vi "Initialize ReadWrite Data.vi"(7 "Name":string, 8 "error in (no error)":errorcluster, 10 "Hardware Output Refs":T1[](array[typedef]) format="%.0x", 11 "Device Ref":T1 format="%.0x") -> (0 "error out":errorcluster, 2 "ReadWrite Data":T2 {"Pairs"."Chan Refs" format="%.0x"}, 3 "Device Ref out":T1=18446744073709551615 format="%.0x")   [LabVIEW 2013, in "FPGA Addon Engine.lvlib" / "Inline Async API.lvlib"]
uses:
  Inline Async API.lvlib
  Controls/ReadWrite Data.ctl
  <vilib>/NI Veristand/Custom Device API/Data Reference.ctl
  <vilib>/NI Veristand/Custom Device API/Custom Device Item Ref.ctl
  <vilib>/NI Veristand/Custom Device API/Data Access Type.ctl
  <vilib>/NI VeriStand/Custom Device API/Custom Device API.lvlib
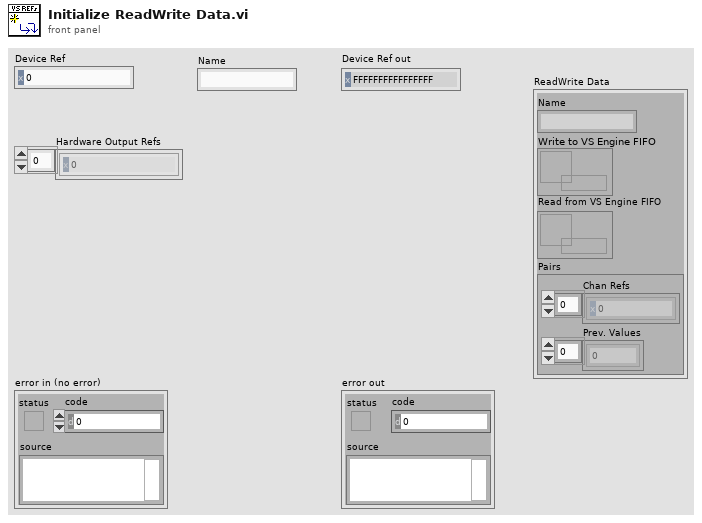
[diagram p1: front panel]
types:
  T1 = typedef "Custom Device API.lvlib/Custom Device Item Ref.ctl" = u64
  T2 = typedef "FPGA Addon Engine.lvlib/Inline Async API.lvlib/ReadWrite Data.ctl" = cluster{"Name":string, "Write to VS Engine FIFO":refnum<k33>, "Read from VS Engine FIFO":refnum<k33>, "Pairs":cluster{"Chan Refs":T3[], "Prev. Values":dbl[]}}
  T3 = typedef "Custom Device API.lvlib/Data Reference.ctl" = i32
  T4 = cluster{"read mode":enum16{"polling", "blocking"}, "write mode":enum16{"polling", "blocking"}}
  T5 = typedef "Custom Device API.lvlib/Data Access Type.ctl" = enum16{"Read", "Write"}
  T6 = typedef "Custom Device API.lvlib/Custom Device Item Info.ctl" = cluster{"Name":string, "Is Channel":bool, "GUID":string, "Is Waveform":bool}
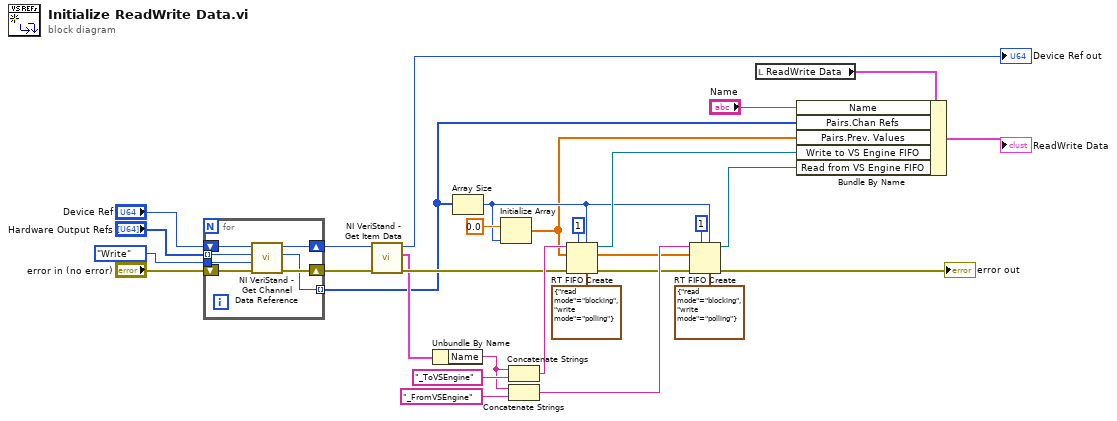
[diagram p0: block diagram]
diagram:
  n1 = for {
    tunnel: "Hardware Output Refs" -> [w32] mode=indexing
    tunnel: Data_Access_Type."Write" ("Access") -> [w31]
    shift-right: [w34] -> w9
    shift-left: "error in (no error)" -> [w35]
    shift-right: [w36] -> w7
    shift-left: "Device Ref" -> [w33]
    tunnel: [w30] -> w3 mode=indexing
    n2 = call <vilib>:"NI VeriStand - Get Channel Data Reference.vi"("error in (no error)"=w35, "Access"=w31, "Channel Ref in"=w32, "Device Ref in"=w33) -> ("error out"=w34:errorcluster, "Channel Data Reference"=w30:T3, "Device Ref out"=w36:T1)  [unwired: 5 in]
  }
  n3 = call <vilib>:"NI VeriStand - Get Item Data.vi"("error in (no error)"=w9, "Item Ref in"=w7) -> ("error out"=w8:errorcluster, "Item Info"=w5:T6, "Item Ref out"=→"Device Ref out":T1)  [unwired: 6 in, 1 out]
  n4 = Unbundle By Name(w5) -> ("Name"=w4:string)
  n5 = Array Size(array=w3) -> (size(s)=w12:i32)
  n6 = Initialize Array(0.0 ("element"), w12) -> (w11:dbl[])
  n7 = Concatenate Strings(w4, "_ToVSEngine" ("string")) -> (w15:string)
  n8 = Concatenate Strings(w4, "_FromVSEngine" ("string")) -> (w14:string)
  n9 = RT FIFO Create(0:w15, 1:w11, 3:w8, 4:u32 1 ("size (10)"), 6:w12, 7:T4 {"read mode"=enum."blocking", "write mode"=enum."polling"} ("r/w modes (polling,polling)")) -> (8:w27:refnum<k33>, 11:w10:errorcluster)  [unwired: 2 in, 1 out]
  n10 = RT FIFO Create(0:w14, 1:w11, 3:w10, 4:u32 1 ("size (10)"), 6:w12, 7:T4 {"read mode"=enum."blocking", "write mode"=enum."polling"} ("r/w modes (polling,polling)")) -> (8:w28:refnum<k33>, 11:→"error out":errorcluster)  [unwired: 2 in, 1 out]
  n11 = local read "ReadWrite Data"() -> (w2:T2)
  n12 = Bundle By Name(cluster=w2, "Name"="Name", "Pairs.Chan Refs"=w3, "Pairs.Prev. Values"=w11, "Write to VS Engine FIFO"=w27, "Read from VS Engine FIFO"=w28) -> (→"ReadWrite Data":T2)
